vi "Calculate Cubic Bezier Point.vi"(7 "t":dbl, 8 "d":dbl, 9 "c":dbl, 10 "b":dbl, 11 "a":dbl) -> (3 "f(t)":dbl)   [LabVIEW 2019, in "Tool Path.lvclass"]
uses:
  Tool Path.lvclass
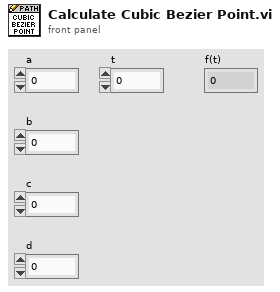
[diagram p1: front panel]
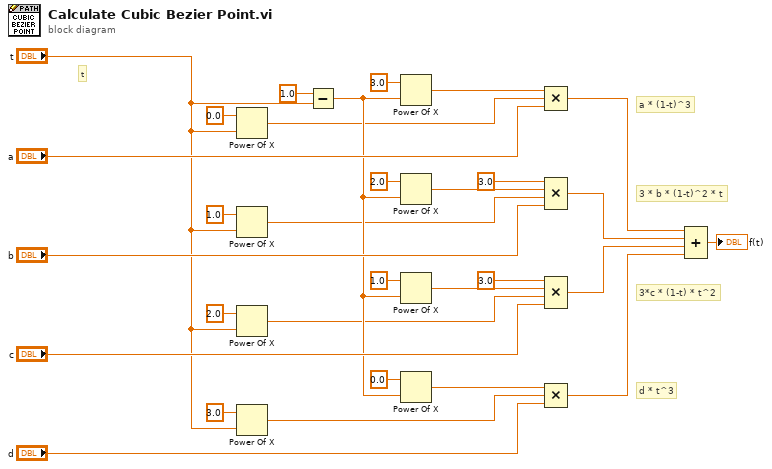
[diagram p0: block diagram]
diagram:
  # "d * t^3"
  # "3*c * (1-t) * t^2"
  # "3 * b * (1-t)^2 * t"
  # "a * (1-t)^3"
  # "t"
  n1 = Power Of X(1:"t", 2:0.0 ("y")) -> (0:w8:dbl)
  n2 = Power Of X(1:"t", 2:1.0 ("y")) -> (0:w14:dbl)
  n3 = Power Of X(1:"t", 2:2.0 ("y")) -> (0:w10:dbl)
  n4 = Power Of X(1:"t", 2:3.0 ("y")) -> (0:w6:dbl)
  n5 = Subtract(x=1.0, y="t") -> (x-y=w24:dbl)
  n6 = Power Of X(1:w24, 2:3.0 ("y")) -> (0:w9:dbl)
  n7 = Power Of X(1:w24, 2:2.0 ("y")) -> (0:w15:dbl)
  n8 = Power Of X(1:w24, 2:1.0 ("y")) -> (0:w11:dbl)
  n9 = Power Of X(1:w24, 2:0.0 ("y")) -> (0:w7:dbl)
  n10 = Compound Arithmetic op=MULTIPLY(w9, w8, "a") -> (w5:dbl)
  n11 = Compound Arithmetic op=MULTIPLY(3.0 ("value"), w15, w14, "b") -> (w4:dbl)
  n12 = Compound Arithmetic op=MULTIPLY(3.0 ("value"), w11, w10, "c") -> (w3:dbl)
  n13 = Compound Arithmetic op=MULTIPLY(w7, w6, "d") -> (w2:dbl)
  n14 = Compound Arithmetic op=ADD(w5, w4, w3, w2) -> (→"f(t)":dbl)
